vi "Rename Any Implemented Method.vi"(8 "error in":errorcluster, 9 "Name":string, 10 "Class To Rename":refnum<vi>) -> (0 "error out":errorcluster)   [LabVIEW 2021, in "_Rename.lvlib" / "SAS.lvlib"]
uses:
  <vilib>/Utility/traverseref.llb/TRef TravTarget.ctl
  SAS.lvlib
  <vilib>/Utility/traverseref.llb/VI Scripting - Traverse.lvlib
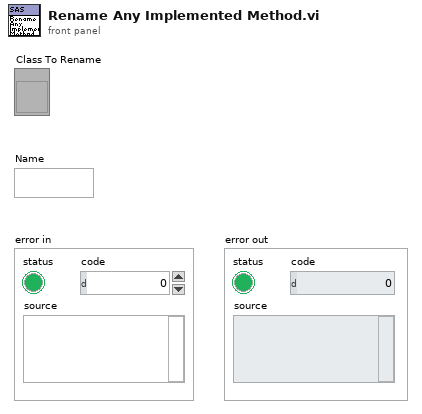
[diagram p1: front panel]
types:
  T1 = typedef "TRef TravTarget.ctl" = enum16{"FP", "BD", "Other"}
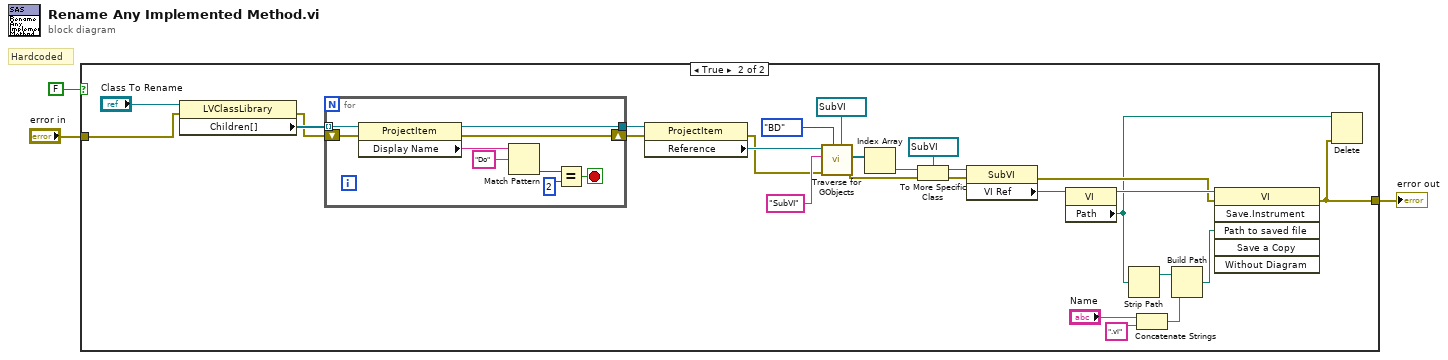
[diagram p0: block diagram]
diagram:
  # "Hardcoded"
  n1 = case shown="True" FALSE {
    tunnel: "error in" -> [w4 w10]
    tunnel: [w4 w9] -> w3
    frame False {
    }
    frame True {
      n2 = property class="LVClassLibrary"(reference="Class To Rename", error in=w10) -> (error out=w15:errorcluster, "Children[]"=w16:refnum<vi>[])  [unwired: 1 out]
      n3 = for {
        tunnel: w16 -> [w40] mode=indexing
        shift-right: [w37] -> w13
        shift-left: w15 -> [w38]
        tunnel: [w36] -> w14
        stop <- w34 stop-if-true
        n4 = property class="ProjectItem"(reference=w40, error in=w38) -> (reference out=w36:refnum<vi>, error out=w37:errorcluster, "Display Name"=w35:string)
        n5 = Match Pattern(string=w35, regular expression="Do") -> (offset past match=w32:i32)  [unwired: 1 in, 3 out]
        n6 = Equal?(x=w32, y=2 ("x")) -> (x = y?=w34:bool)
      }
      n7 = property class="ProjectItem"(reference=w14, error in=w13) -> (error out=w11:errorcluster, "Reference"=w12:refnum<vi>)  [unwired: 1 out]
      n8 = call <vilib>:"Traverse for GObjects.vi"("Other Refnum"=refnum<vi> refnum, "Traverse Target"=TRef_TravTarget."BD", "error in (no error)"=w11, "Class Name"="SubVI", "VI Refnum"=w12) -> ("error out"=w29:errorcluster, "References"=w28:refnum<vi>[])  [unwired: 3 in, 2 out]
      n9 = Index Array(array=w28) -> (element=w26:refnum<vi>)  [unwired: 1 in]
      n10 = To More Specific Class(target class=refnum<vi> refnum ("Other Refnum"), reference=w26, error in=w29) -> (specific class reference=w25:refnum<vi>, error out=w27:errorcluster)
      n11 = property class="SubVI"(reference=w25, error in=w27) -> (error out=w19:errorcluster, "VI Ref"=w23:refnum<vi>)  [unwired: 1 out]
      n12 = property class="VI"(reference=w23) -> (reference out=w22:refnum<vi>, "Path"=w8:path)  [unwired: 1 in, 1 out]
      n13 = Strip Path(path=w8) -> (stripped path=w21:path)  [unwired: 1 out]
      n14 = Concatenate Strings("Name", ".vi" ("string")) -> (w17:string)
      n15 = Build Path(base path=w21, name or relative path=w17) -> (appended path=w20:path)
      n16 = invoke class="VI" method="Save.Instrument"(reference=w22, error in=w19, "Path to saved file"=w20) -> (error out=w9:errorcluster)  [unwired: 3 in, 5 out]
      n17 = Delete(path (use dialog)=w8, error in=w9) -> ()  [unwired: 3 in, 3 out]
    }
  }
  "error out" <- w3
